vi "CSDB_Transfer.main.vi"() -> ()   [LabVIEW 2014, in "CSDB_Transfer.lvlib"]
doc: "Converts database entries of instances to ini files and vice versa."
uses:
  CSDB_Transfer.lvlib
  CSDB_Common/CSDB_Common.lvlib
panel:
  in  "Tab Control":enum32{"INI --> DB", "DB --> INI"}(tab)=enum."DB --> INI"
  in  "select inifile":path
  in  "INI 2 DB":bool
  in  "Included Data":i32(listbox)
  in  "Included Instances":i32(listbox)
  in  "create \ntag-file":bool
  in  "add multiple":bool
  in  "match pattern":string
  in  "clear":bool
  in  "Instance":u16(ring) items=["AFG1", "AFG2", "AFG3", "AFG4", "AFG5", "AFG6", "AG33XXX_1", "AG33XXX_2", "AnalogHVGOG", "AnalogHV\\Super", "CAN0", "CAN1", "CANTestGOG", "CANTest\\Super", "CSTestGUI", "DG535Test", "DIO_PB0", "DIO_PB1", "DIO_PB2", "DIO_PB3", "DIO_PB4", "DIO_PB5", "DIO_PB6", "DIO_PB7", "DSCAlarm", "DSCAlarm1", "DSCBackend\\Super", "DSCInterface", "DSCInterfaceTest", "DSCTrend", "DiscArchiver", "EHQ0", "EHQSim0", "EventBuilder", "HVSwitch0", "HVSwitch1", "HVSwitch2", "HVSwitchesGOG", "HVSwitches\\Super", "HV_PB_Vorort0", "HV_PB_Vorort1", "HV_PB_Vorort2", "HV_PB_Vorort3", "HV_PB_Vorort4", "HV_PB_Vorort5", "Labor2\\Super", "LxTest\\Super", "MCS", "MIOCounter", "MIOE_AIO", "MIOE_DIO", "MIOE_Scope", "MM6Archiver", "MMLebit", "MassMeas", "OPCGateway2", "OPCGateway\\Super", "OPCInterface", "Office11\\Super", "Office9\\Super", "PB_DIOGOG", "PB_DIO\\Super", "R_PB0", "R_PB1", "SR430GOG", "STTest\\Super", "SimAFG", "SimDigiIO", "SimMCS", "SimPowerSupply", "SimTG", "TDS224", "TestDPS", "TestSystem71\\Super", "TestSystem\\Super", "USBCam2", "Vorort1\\Super", "Vorort20\\Super", "Vorort2\\Super", "Vorort4\\Super", "Vorort6\\Super", "Vorort6b\\Super", "VorortCam", "VorortCam\\Super", "test1", "test2", "test3", "test4", "test5", "testPBPS"]
  in  "DB 2 INI":bool
  in  "Data":i32(listbox)
  in  "Instances":i32(listbox)
  in  "add":bool
  in  "exit":bool
  in  "Database":string="Process"
  # "INI ---> DB"
  # "DB ---> INI"
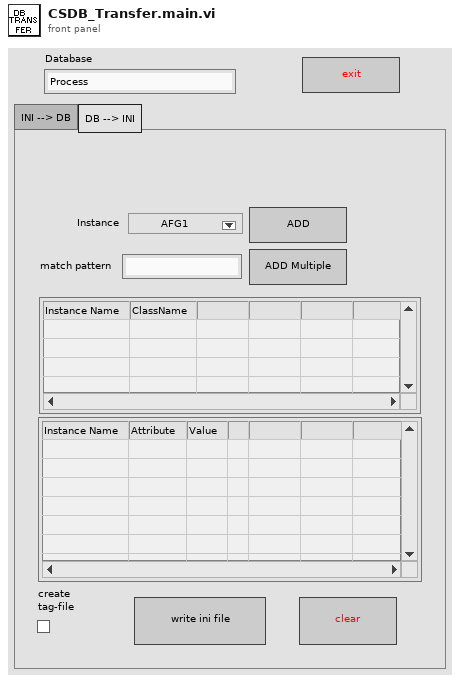
[diagram p1: front panel]
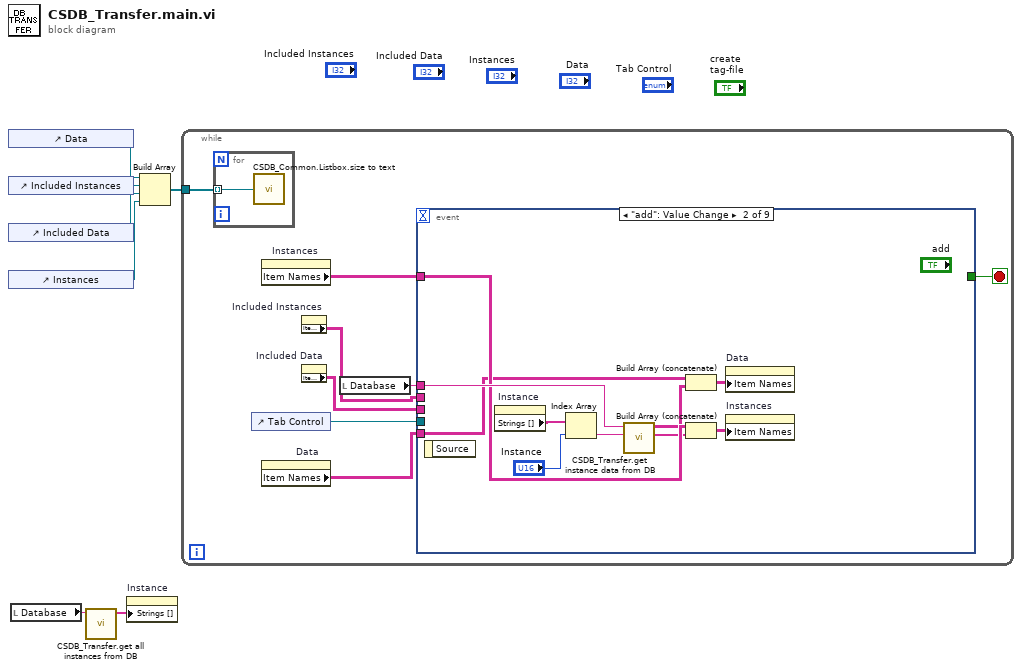
[diagram p0: block diagram]
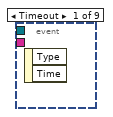
[diagram p2: hidden frame]
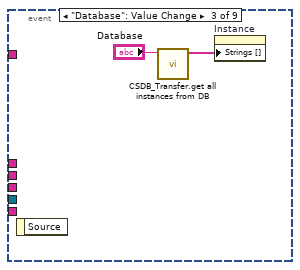
[diagram p3: hidden frame]
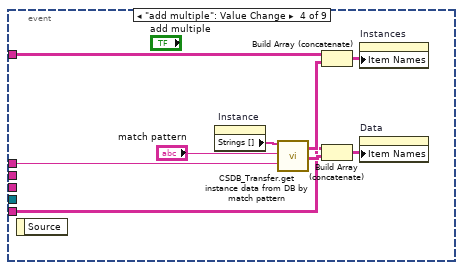
[diagram p4: hidden frame]
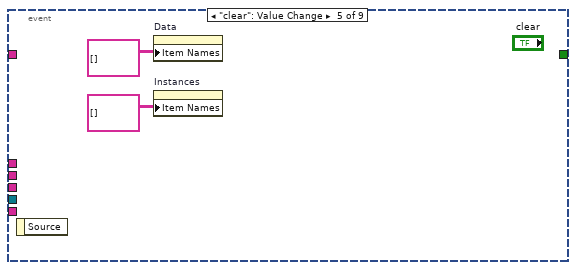
[diagram p5: hidden frame]
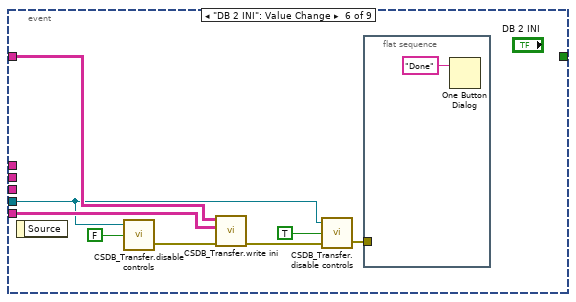
[diagram p6: hidden frame]
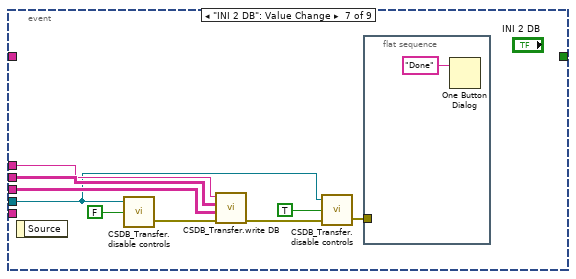
[diagram p7: hidden frame]
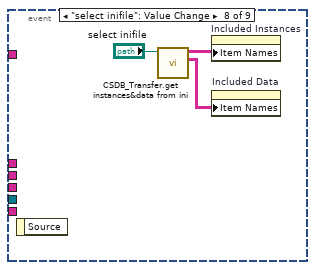
[diagram p8: hidden frame]
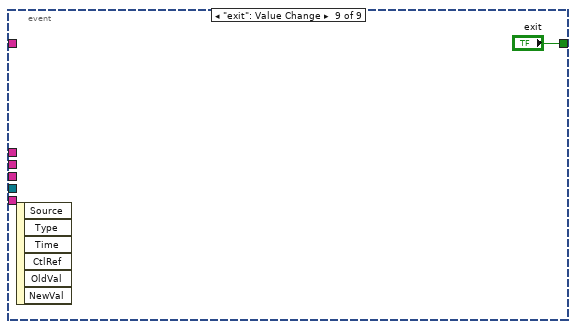
[diagram p9: hidden frame]
diagram:
  n1 = control-ref of="Data"() -> (w5:refnum<vi>)
  n2 = control-ref of="Included Instances"() -> (w4:refnum<vi>)
  n3 = control-ref of="Included Data"() -> (w3:refnum<vi>)
  n4 = control-ref of="Instances"() -> (w2:refnum<vi>)
  n5 = local read "Database"() -> (w7:string)
  n6 = call "CSDB_Transfer.get all instances from DB.vi"("Data Source"=w7) -> ("sorted array"=w6:string[])  [unwired: 5 in, 1 out]
  n7 = property on="Instance" class="Ring (strict)"("Strings []"=w6) -> ()  [unwired: 2 in, 2 out]
  n8 = Build Array(w5, w4, w3, w2) -> (w1:refnum<vi>[])
  n9 = while {
    tunnel: w1 -> [w8]
    stop <- w15 stop-if-true
    n10 = for {
      tunnel: w8 -> [w16] mode=indexing
      n11 = call "CSDB_Common.Listbox.size to text.vi"("listbox ref"=w16) -> ()  [unwired: 2 in]
    }
    n12 = control-ref of="Tab Control"() -> (w11:refnum<vi>)
    n13 = property on="Instances" class="MCListbox (strict)"() -> ("Item Names"=w9:string[][])  [unwired: 2 in, 2 out]
    n14 = property on="Data" class="MCListbox (strict)"() -> ("Item Names"=w10:string[][])  [unwired: 2 in, 2 out]
    n15 = property on="Included Instances" class="MCListbox (strict)"() -> ("Item Names"=w12:string[][])  [unwired: 2 in, 2 out]
    n16 = property on="Included Data" class="MCListbox (strict)"() -> ("Item Names"=w13:string[][])  [unwired: 2 in, 2 out]
    n17 = local read "Database"() -> (w14:string)
    n18 = event shown="[1] \"add\": Value Change" {
      selector: _ -> [_ _ _ _ _ _ _ _ _]
      dyn-events: _ -> [_ _ _ _ _ _ _ _ _]
      timeout: _ -> [_ _ _ _ _ _ _ _ _]
      tunnel: [_ _ _ _ _ _ _ _ "exit"] -> w15
      tunnel: w14 -> [_ w26 _ w36 _ _ w50 _ _]
      tunnel: w13 -> [_ _ _ _ _ _ w52 _ _]
      tunnel: w12 -> [_ _ _ _ _ _ w51 _ _]
      tunnel: w11 -> [_ _ _ _ _ w40 w49 _ _]
      tunnel: w10 -> [_ w21 _ w31 _ w43 _ _ _]
      tunnel: w9 -> [_ w22 _ w32 _ w42 _ _ _]
      event Timeout {
        n19 = event-data() -> ()  [unwired: 1 in, 2 out]
      }
      event "add": Value Change {
        n20 = event-data() -> ()  [unwired: 1 in, 1 out]
        n21 = property on="Instance" class="Ring (strict)"() -> ("Strings []"=w25:string[])  [unwired: 2 in, 2 out]
        n22 = Index Array(array=w25, index="Instance") -> (element=w23:string)
        n23 = call "CSDB_Transfer.get instance data from DB.vi"("Instance"=w23, "Data source"=w26) -> ("from DB instance"=w17:string[], "from DB data"=w20:string[][])  [unwired: 3 in, 1 out]
        n24 = Build Array (concatenate)(w21, w20) -> (w19:string[][])
        n25 = Build Array (concatenate)(w22, w17) -> (w18:string[][])
        n26 = property on="Data" class="MCListbox (strict)"("Item Names"=w19) -> ()  [unwired: 2 in, 2 out]
        n27 = property on="Instances" class="MCListbox (strict)"("Item Names"=w18) -> ()  [unwired: 2 in, 2 out]
      }
      event "Database": Value Change {
        n28 = event-data() -> ()  [unwired: 1 in, 1 out]
        n29 = call "CSDB_Transfer.get all instances from DB.vi"("Data Source"="Database") -> ("sorted array"=w27:string[])  [unwired: 5 in, 1 out]
        n30 = property on="Instance" class="Ring (strict)"("Strings []"=w27) -> ()  [unwired: 2 in, 2 out]
      }
      event "add multiple": Value Change {
        n31 = event-data() -> ()  [unwired: 1 in, 1 out]
        n32 = property on="Instance" class="Ring (strict)"() -> ("Strings []"=w37:string[])  [unwired: 2 in, 2 out]
        n33 = call "CSDB_Transfer.get instance data from DB by match pattern.vi"("all instances"=w37, "match pattern"="match pattern", "Data source"=w36) -> ("Instances"=w34:string[][], "data"=w33:string[][])  [unwired: 14 in, 1 out]
        n34 = Build Array (concatenate)(w32, w34) -> (w30:string[][])
        n35 = Build Array (concatenate)(w31, w33) -> (w29:string[][])
        n36 = property on="Instances" class="MCListbox (strict)"("Item Names"=w30) -> ()  [unwired: 2 in, 2 out]
        n37 = property on="Data" class="MCListbox (strict)"("Item Names"=w29) -> ()  [unwired: 2 in, 2 out]
      }
      event "clear": Value Change {
        n38 = event-data() -> ()  [unwired: 1 in, 1 out]
        n39 = property on="Data" class="MCListbox (strict)"("Item Names"=string[][] []) -> ()  [unwired: 2 in, 2 out]
        n40 = property on="Instances" class="MCListbox (strict)"("Item Names"=string[][] []) -> ()  [unwired: 2 in, 2 out]
      }
      event "DB 2 INI": Value Change {
        n41 = event-data() -> ()  [unwired: 1 in, 1 out]
        n42 = call "CSDB_Transfer.disable controls.vi"("on / off"=FALSE, "Tab Control"=w40) -> ("error out"=w44:errorcluster)  [unwired: 2 in]
        n43 = call "CSDB_Transfer.write ini.vi"("error in"=w44, "db2ini data"=w43, "db2ini instances"=w42) -> ("error out"=w41:errorcluster)  [unwired: 4 in]
        n44 = call "CSDB_Transfer.disable controls.vi"("error in (no error)"=w41, "on / off"=TRUE, "Tab Control"=w40) -> ("error out"=w47:errorcluster)  [unwired: 1 in]
        n45 = flat-sequence {
          tunnel: w47 -> [_]
          frame #0 {
            n46 = One Button Dialog(message="Done") -> ()  [unwired: 1 in, 1 out]
          }
        }
      }
      event "INI 2 DB": Value Change {
        n47 = event-data() -> ()  [unwired: 1 in, 1 out]
        n48 = call "CSDB_Transfer.disable controls.vi"("on / off"=FALSE, "Tab Control"=w49) -> ("error out"=w53:errorcluster)  [unwired: 2 in]
        n49 = call "CSDB_Transfer.write DB.vi"("error in (no error)"=w53, "Data array"=w52, "Instances & Classes"=w51, "Data source"=w50) -> ("error out"=w55:errorcluster)  [unwired: 3 in]
        n50 = call "CSDB_Transfer.disable controls.vi"("error in (no error)"=w55, "on / off"=TRUE, "Tab Control"=w49) -> ("error out"=w54:errorcluster)  [unwired: 1 in]
        n51 = flat-sequence {
          tunnel: w54 -> [_]
          frame #0 {
            n52 = One Button Dialog(message="Done") -> ()  [unwired: 1 in, 1 out]
          }
        }
      }
      event "select inifile": Value Change {
        n53 = event-data() -> ()  [unwired: 1 in, 1 out]
        n54 = call "CSDB_Transfer.get instances&data from ini.vi"("configuration file path"="select inifile") -> ("from ini data"=w60:string[][], "from ini instances"=w59:string[][])  [unwired: 4 in, 1 out]
        n55 = property on="Included Instances" class="MCListbox (strict)"("Item Names"=w59) -> ()  [unwired: 2 in, 2 out]
        n56 = property on="Included Data" class="MCListbox (strict)"("Item Names"=w60) -> ()  [unwired: 2 in, 2 out]
      }
      event "exit": Value Change {
        n57 = event-data() -> ()  [unwired: 1 in, 6 out]
      }
    }
  }
